vi "pulse detector.vi"(4 "calculate timeing inside":bool, 6 "time":u64, 9 "reciver_params":T1, 10 "IQ sampels":u32, 11 "input valid":bool) -> (2 "output valid":bool, 3 "data out":u64[](array[numeric]))   [LabVIEW 2021]
uses:
  FPGA/reciver params.ctl
panel:
  # "PDW: 2*64\nF - 16 (index)\nPW - 16 (fft cycles)\nAMP - 32 (number)\nTend -64 (fft cycles)"
  # "2*i16 (i,q) combind to u32"
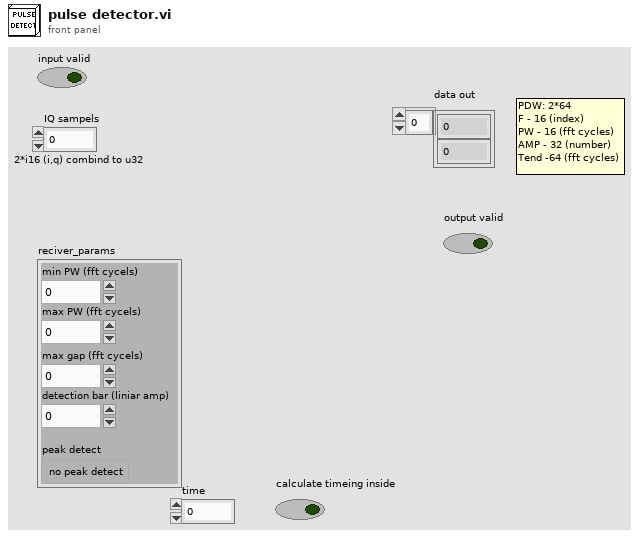
[diagram p1: front panel]
types:
  T1 = typedef "reciver params.ctl" = cluster{"min PW (fft cycels)":u16, "max PW (fft cycels)":u16, "max gap (fft cycels)":u8, "detection bar (liniar amp)":fxp<+,64,63>, "peak detect":bool}
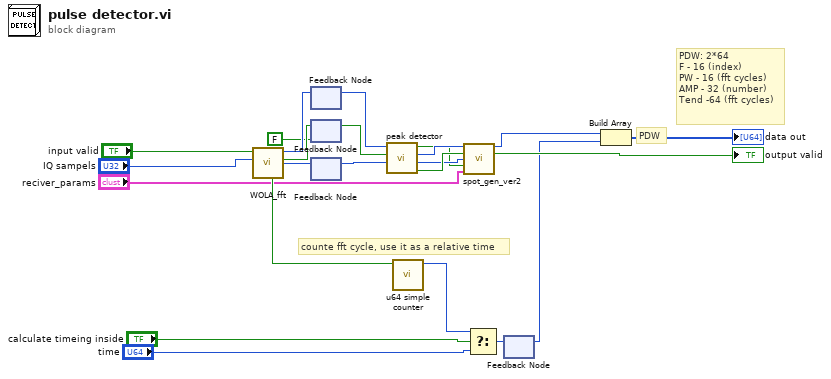
[diagram p0: block diagram]
diagram:
  # "PDW: 2*64\nF - 16 (index)\nPW - 16 (fft cycles)\nAMP - 32 (number)\nTend -64 (fft cycles)"
  # "PDW"
  # "counte fft cycle, use it as a relative time"
  n1 = call "WOLA_fft.vi"("data in"="IQ sampels", "input valid"="input valid") -> ("data index"=w9:u16, "output valid"=w11:bool, "fft_output"=w12:u64, "new fft cycle"=w13:bool)  [unwired: 6 in]
  n2 = feedback #1() -> (w8:u64)  [unwired: 1 in]
  n3 = feedback-in #1(w12) -> ()
  n4 = feedback #2(FALSE ("output valid 2")) -> (w7:bool)
  n5 = feedback-in #2(w11) -> ()
  n6 = feedback #3() -> (w6:u16)  [unwired: 1 in]
  n7 = feedback-in #3(w9) -> ()
  n8 = call "peak detector.vi"("data index"=w6, "output valid in"=w7, "fft_output"=w8) -> ("output valid"=w4:bool, "adress"=w3:u16, "amplitude"=w5:u32, "peak"=w2:bool)  [unwired: 5 in]
  n9 = call "u64 simple counter.vi"("new fft cycle"=w13) -> ("value"=w18:u64)  [unwired: 10 in]
  n10 = call "spot_gen_ver2.vi"("amp"=w5, "input valid"=w4, "data index"=w3, "peak"=w2, "reciver_params"="reciver_params") -> ("PDW"=w23:u64, "output valid"=→"output valid":bool)  [unwired: 8 in, 1 out]
  n11 = Select(t=w18, s="calculate timeing inside", f="time") -> (s? t:f=w15:u64)
  n12 = feedback-in #4(w15) -> ()
  n13 = feedback #4() -> (w14:u64)  [unwired: 1 in]
  n14 = Build Array(w23, w14) -> (→"data out":u64[])
